vi "Bring Window To Front.vi"(8 "error in (no error)":errorcluster, 11 "Window Name":string) -> (0 "error out":errorcluster, 2 "Handle":dbl, 3 "Error":i32)   [LabVIEW 2024]
doc: "This VI will programmatically move a window to the front whether its a LabVIEW window or not."
uses:
  user32.dll
panel:
  # "Overview: This VI will programmatically move a window to the front whether its a LabVIEW window or not.\nRequirements: LabVIEW 2012 (or compatible)\nInstructions: \n1. Choose the window name you want to bring to front\n2. Run the VI\n3. Stop Execution"
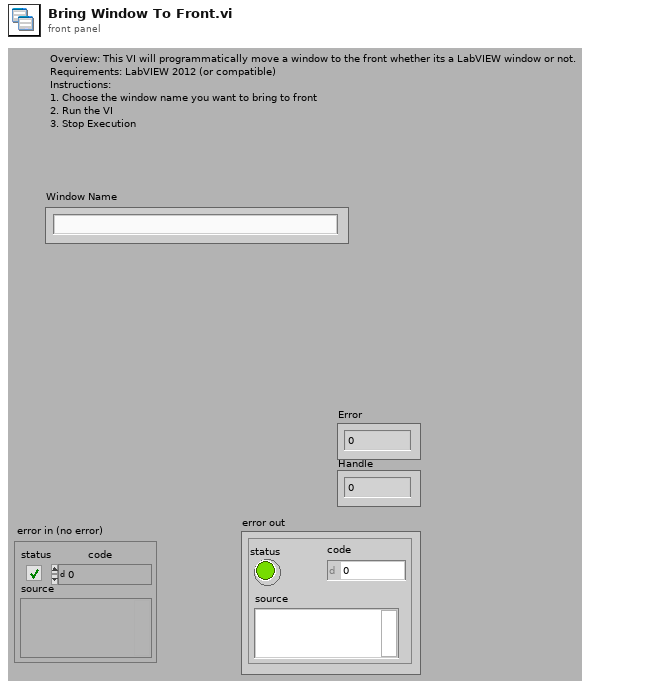
[diagram p1: front panel]
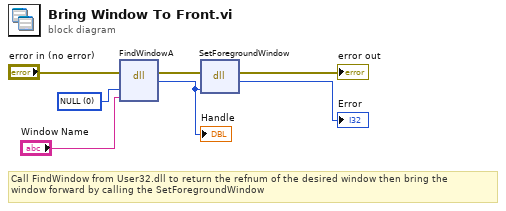
[diagram p0: block diagram]
diagram:
  w6 = 0 items=["NULL"]
  # "Call FindWindow from User32.dll to return the refnum of the desired window then bring the \nwindow forward by calling the SetForegroundWindow"
  n1 = dll-call lib="user32.dll" fn="FindWindowA" label="FindWindow"(error in="error in (no error)", "lpszClassName"=w6, "lpszWindowName"="Window Name") -> (error out=w7:errorcluster, "hWnd"=w5:u32)  [unwired: 3 in, 2 out]
  "Handle" <- w5
  n2 = dll-call lib="user32.dll" fn="SetForegroundWindow"(error in=w7, "Handle"=w5) -> (error out=→"error out":errorcluster, "return type"=→"Error":i32)  [unwired: 3 in, 1 out]
